vi "Receive A Frame.vi"(8 "error in (no error)":errorcluster, 11 "Receiver in":refnum<class "Receiver.lvclass">) -> (0 "error out":errorcluster, 2 "Received data":i32[](array[numeric]), 3 "Receiver out":refnum<class "Receiver.lvclass">)   [LabVIEW 2013, in "Receiver.lvclass"]
uses:
  Receiver.lvclass
  Receiver.lvclass/Receiver.ctl
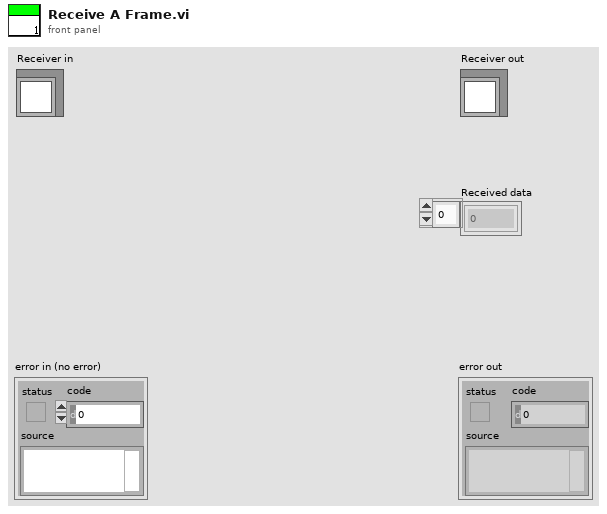
[diagram p1: front panel]
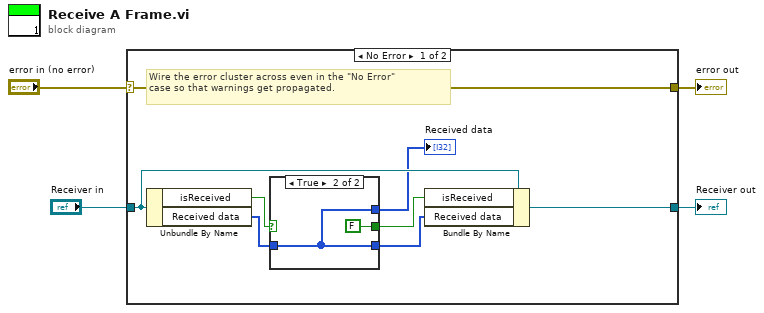
[diagram p0: block diagram]
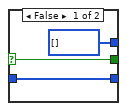
[diagram p2: hidden frame]
diagram:
  n1 = case shown="No Error" "error in (no error)" {
    selector: "error in (no error)" -> [w12 w19]
    tunnel: [w12 w19] -> w3
    tunnel: [w10 w18] -> w1
    tunnel: "Receiver in" -> [w11 w18]
    frame No Error {
      # "Wire the error cluster across even in the \"No Error\"\ncase so that warnings get propagated."
      n2 = Unbundle By Name(w11) -> ("isReceived"=w9:bool, "Received data"=w7:i32[])
      n3 = case shown="True" w9 {
        selector: w9 -> [w15 _]
        tunnel: [w14 w16] -> w8
        tunnel: w7 -> [w14 w16]
        tunnel: [w15 FALSE] -> w6
        tunnel: [i32[] [] ("Received data") w16] -> w5
        frame False {
        }
        frame True {
        }
      }
      "Received data" <- w5
      n4 = Bundle By Name(cluster=w11, "isReceived"=w6, "Received data"=w8) -> (w10:refnum<class "Receiver.lvclass">)
    }
    frame Error {
    }
  }
  "error out" <- w3
  "Receiver out" <- w1
